vi "Actor Core.vi"(8 "error in":errorcluster, 11 "Assert Display in":refnum<class "Assert Display.lvclass">) -> (0 "error out":errorcluster, 3 "Actor out":refnum<class "Actor.lvclass">)   [LabVIEW 2016, in "Assert API Components.lvlib" / "Assert Display.lvlib" / "Assert Display.lvclass"]
doc: "(<B>Filename</B>: Actor Framework.lvlib:Actor.lvclass:Actor Core.vi)\n\nReceives messages to the actor, reacts to them, and initiates any error handling that may shut the actor down.\n\nDescendant classes may override this VI to append parallel tasks for the actor to complete while it handles messages. Overrides use the Call Parent Method node."
uses:
  Assert Display.lvclass
  C:/Program Files (x86)/National Instruments/LabVIEW 2016/vi.lib/ActorFramework/Actor/Actor.lvclass
  C:/Users/ukhornp/Documents/Projects/actor_assert_api/Core/Base UI Actor/Base UI Actor/Base UI Actor.lvclass
  <vilib>/ActorFramework/Actor/Actor.lvclass
  Filter Config Display/Filter Config Display/Filter Config Display.lvclass
  C:/Users/ukhornp/Documents/Projects/actor_assert_api/Core/Base UI Component/Base UI Component/Base UI Component.lvclass
  Main Display/Main Display/Main Display.lvclass
  Service Config Display/Service Config Display/Service Config Display.lvclass
  Assert Display.lvclass/Assert Display.ctl
  Base UI Actor/Base UI Actor/Base UI Actor.lvclass/Base UI Actor.ctl
  <vilib>/ActorFramework/Actor/Actor.lvclass/Actor.ctl
  <vilib>/ActorFramework/Message Enqueuer/Message Enqueuer.lvclass/Message Enqueuer.ctl
  Assert Display Messages/Change Screen Msg/Change Screen Msg.lvclass/Change Screen Msg.ctl
  <vilib>/ActorFramework/Message Enqueuer/Init from Existing Queue.vi
  <vilib>/ActorFramework/Message Enqueuer/Enqueue.vi
  <vilib>/ActorFramework/Stop Msg/Stop Msg.lvclass
  C:/Program Files (x86)/National Instruments/LabVIEW 2016/vi.lib/ActorFramework/Message/Message.lvclass
  Assert Display Messages/Change Screen Msg/Change Screen Msg.lvclass
  <vilib>/Utility/LVClass/Get LV Class Name.vi
  <resource>/AFDebug/Generate Trace for Message.vi
  <vilib>/ActorFramework/Message Priority Queue/Priority Enqueue.vi
  <vilib>/ActorFramework/Message Enqueuer/Message Enqueuer.lvclass
  Base UI Actor/Base UI Actor/Base UI Actor.lvclass
  Base UI Component/Base UI Component/Base UI Component.lvclass
panel:
  in  "Filters":bool
  in  "Services":bool
  in  "Main":bool
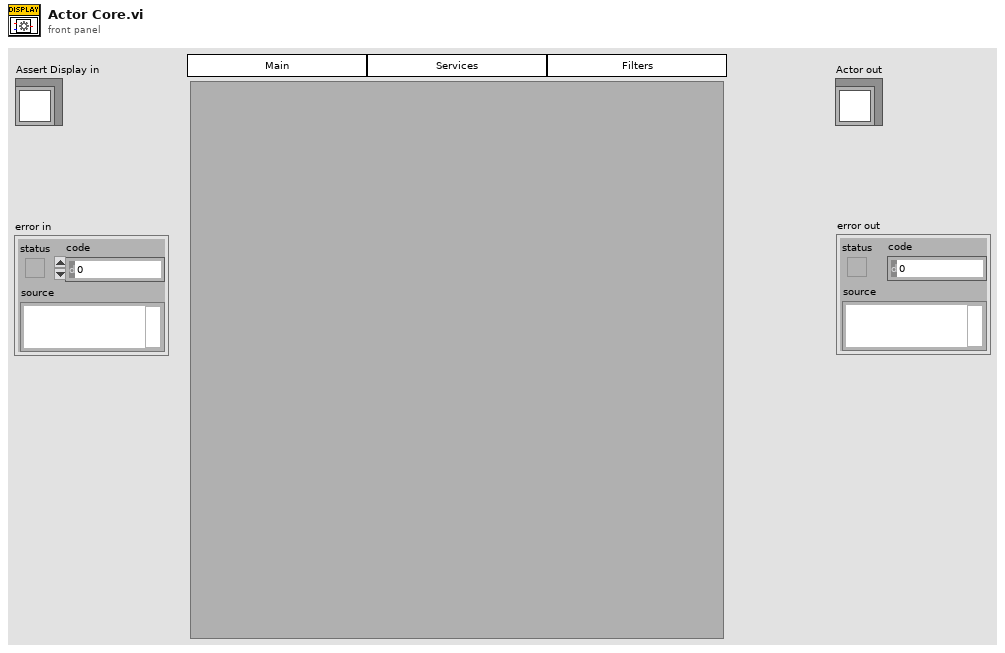
[diagram p1: front panel]
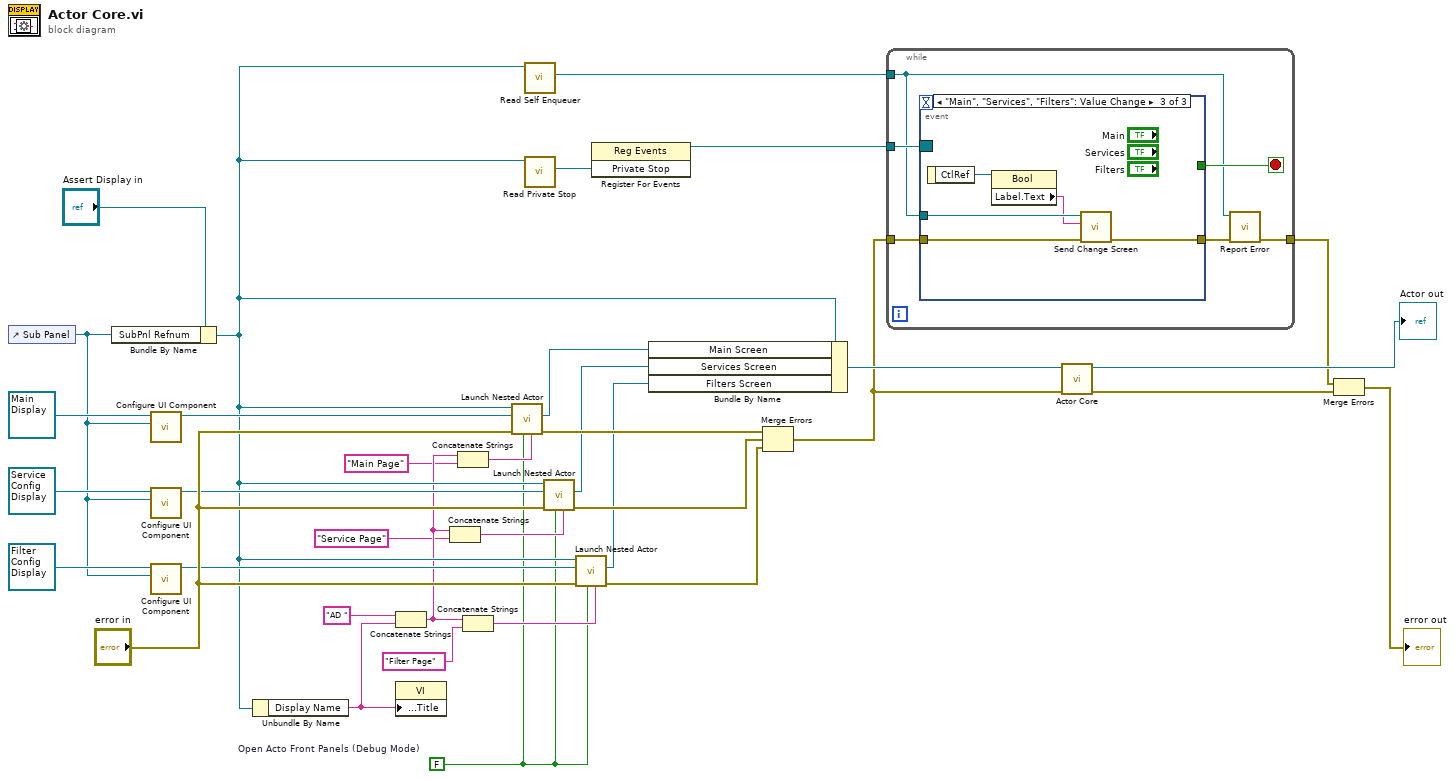
[diagram p0: block diagram]
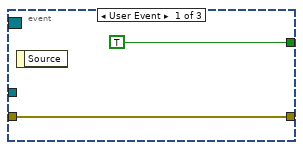
[diagram p2: hidden frame]
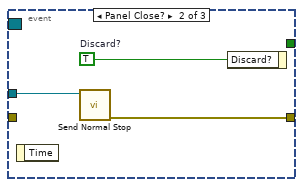
[diagram p3: hidden frame]
diagram:
  w1 = FALSE  # Open Acto Front Panels (Debug Mode)
  n1 = control-ref of="Sub Panel"() -> (w12:refnum<vi>)
  n2 = Bundle By Name(cluster="Assert Display in", "SubPnl Refnum"=w12) -> (w11:refnum<class "Assert Display.lvclass">)
  n3 = call "Configure UI Component.vi"("SubPanel Reference"=w12, "Base UI Component in"=refnum<class "Main Display.lvclass"> refnum ("Assert Display.lvlib:Main Display.lvlib:Main Display.lvclass")) -> ("Base UI Component out"=w15:refnum<class "Main Display.lvclass">)  [unwired: 9 in]
  n4 = call "Configure UI Component.vi"("SubPanel Reference"=w12, "Base UI Component in"=refnum<class "Service Config Display.lvclass"> refnum ("Assert Display.lvlib:Service Config Display.lvlib:Service Config Display.lvclass")) -> ("Base UI Component out"=w14:refnum<class "Service Config Display.lvclass">)  [unwired: 9 in]
  n5 = call "Configure UI Component.vi"("SubPanel Reference"=w12, "Base UI Component in"=refnum<class "Filter Config Display.lvclass"> refnum ("Assert Display.lvlib:Filter Config Display.lvlib:Filter Config Display.lvclass")) -> ("Base UI Component out"=w13:refnum<class "Filter Config Display.lvclass">)  [unwired: 9 in]
  n6 = Unbundle By Name(w11) -> ("Display Name"=w2:string)
  n7 = Concatenate Strings("AD " ("string"), w2) -> (w9:string)
  n8 = property class="VI"("Front Panel.Title"=w2) -> ()  [unwired: 2 in, 2 out]
  n9 = Concatenate Strings(w9, "Service Page" ("string")) -> (w3:string)
  n10 = Concatenate Strings(w9, "Main Page" ("string")) -> (w4:string)
  n11 = Concatenate Strings(w9, "Filter Page" ("string")) -> (w7:string)
  n12 = call <vilib>:"Launch Nested Actor.vi"("Debug Alias"=w4, "Open Actor Core front panel? (F)"=w1, "error in (no error)"="error in", "Nested Actor"=w15, "Caller Actor in"=w11) -> ("error out"=w25:errorcluster, "Nested Actor's Enqueuer"=w21:refnum<class "Message Enqueuer.lvclass">)  [unwired: 4 in, 1 out]
  n13 = call <vilib>:"Read Self Enqueuer.vi"("Actor"=w11) -> ("Self Enqueuer"=w31:refnum<class "Message Enqueuer.lvclass">)  [unwired: 10 in]
  n14 = call "Read Private Stop.vi"("Base UI Actor in"=w11) -> ("Private Stop"=w33:refnum<user-event>)  [unwired: 10 in]
  n15 = call <vilib>:"Launch Nested Actor.vi"("Debug Alias"=w3, "Open Actor Core front panel? (F)"=w1, "error in (no error)"="error in", "Nested Actor"=w14, "Caller Actor in"=w11) -> ("error out"=w24:errorcluster, "Nested Actor's Enqueuer"=w20:refnum<class "Message Enqueuer.lvclass">)  [unwired: 4 in, 1 out]
  n16 = call <vilib>:"Launch Nested Actor.vi"("Debug Alias"=w7, "Open Actor Core front panel? (F)"=w1, "error in (no error)"="error in", "Nested Actor"=w13, "Caller Actor in"=w11) -> ("error out"=w23:errorcluster, "Nested Actor's Enqueuer"=w19:refnum<class "Message Enqueuer.lvclass">)  [unwired: 4 in, 1 out]
  n17 = register-events(w33) -> (reference out=w32:refnum<event-registration>)  [unwired: 2 in, 1 out]
  n18 = Bundle By Name(cluster=w11, "Main Screen"=w21, "Services Screen"=w20, "Filters Screen"=w19) -> (w22:refnum<class "Assert Display.lvclass">)
  n19 = Merge Errors(w25, w24, w23) -> (w18:errorcluster)
  n20 = while {
    tunnel: w32 -> [w41]
    tunnel: w31 -> [w36]
    tunnel: w18 -> [w39]
    tunnel: [w37] -> w16
    stop <- w40 stop-if-true
    n21 = event shown="[2] \"Main\", \"Services\", \"Filters\": Value Change" {
      selector: w41 -> [_ _ _]
      dyn-events: _ -> [_ _ _]
      timeout: _ -> [_ _ _]
      tunnel: [TRUE _ _] -> w40
      tunnel: w36 -> [_ w45 w51]
      tunnel: w39 -> [w42 _ w48]
      tunnel: [w42 w44 w47] -> w38
      event User Event {
        n22 = event-data() -> ()  [unwired: 1 in, 1 out]
      }
      event Panel Close? {
        w46 = TRUE  # Discard?
        n23 = event-data() -> ()  [unwired: 1 in, 1 out]
        n24 = call <vilib>:"Send Normal Stop.vi"("Message Enqueuer"=w45) -> ("error out"=w44:errorcluster)  [unwired: 10 in]
        n25 = event-data("Discard?"=w46) -> ()  [unwired: 1 in, 1 out]
      }
      event "Main", "Services", "Filters": Value Change {
        n26 = event-data() -> ("CtlRef"=w50:refnum<vi>)  [unwired: 1 in]
        n27 = property class="Bool"(reference=w50) -> ("Label.Text"=w49:string)  [unwired: 1 in, 2 out]
        n28 = call "Send Change Screen.vi"("error in (no error)"=w48, "Screen"=w49, "Message Enqueuer"=w51) -> ("error out"=w47:errorcluster)  [unwired: 7 in, 1 out]
      }
    }
    n29 = call "Report Error.vi"("error in (no error)"=w38, "Self Enqueuer"=w36) -> ("error out"=w37:errorcluster)  [unwired: 9 in]
  }
  n30 = call-parent "Actor Core.vi"("error in"=w18, "Actor in"=w22) -> ("error out"=w35:errorcluster, "Actor out"=→"Actor out":refnum<class "Actor.lvclass">)  [unwired: 8 in]
  n31 = Merge Errors(w16, w35) -> (→"error out":errorcluster)
